vi "Write Subdiagram Labels.vi"(8 "Error In":errorcluster, 11 "DisableStructure In":refnum<vi>) -> (0 "Error Out":errorcluster, 3 "DisableStructure Out":refnum<vi>)   [LabVIEW 2017, in "Toolkit VIs.lvlib"]
uses:
  Toolkit VIs.lvlib
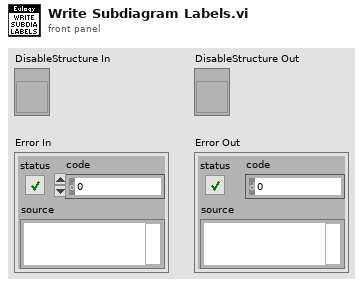
[diagram p1: front panel]
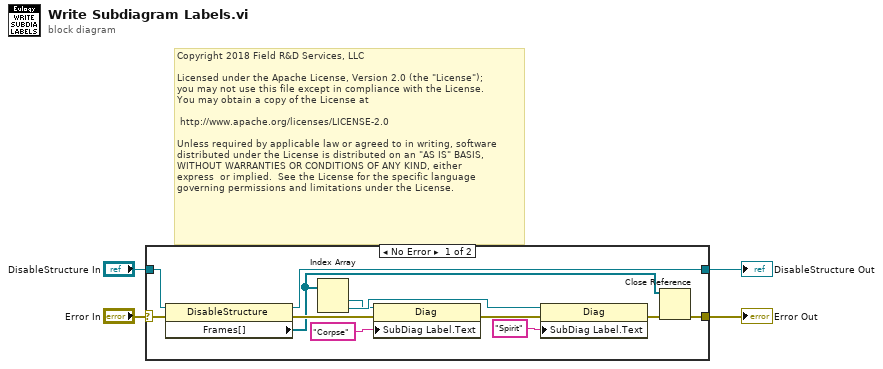
[diagram p0: block diagram]
diagram:
  # "Copyright 2018 Field R&D Services, LLC\n\nLicensed under the Apache License, Version 2.0 (the \"License\");\nyou may not use this file except in compliance with the License.\nYou may obtain a copy of the License at\n\n\thttp://www.apache.org/licenses/LICENSE-2.0\n\nUnless required by applicable law or agreed to in writing, software\ndistributed under the License is distributed on an \"AS IS\" BASIS,\nWITHOUT WARRANTIES OR CONDITIONS OF ANY KIND, either \nexpress  or implied.  See the License for the specific language \ngoverning permissions and limitations under the License."
  n1 = case shown="No Error" "Error In" {
    selector: "Error In" -> [w8 w17]
    tunnel: [w7 w17] -> w4
    tunnel: [w16 w18] -> w3
    tunnel: "DisableStructure In" -> [w10 w18]
    frame No Error {
      n2 = property class="DisableStructure"(reference=w10, error in=w8) -> (reference out=w16:refnum<vi>, error out=w9:errorcluster, "Frames[]"=w5:refnum<vi>[])
      n3 = Index Array(array=w5) -> (element #1=w12:refnum<vi>, element #2=w14:refnum<vi>)  [unwired: 2 in]
      n4 = property class="Diag"(reference=w12, error in=w9, "SubDiag Label.Text"="Corpse" ("Subdiagram Label.Text")) -> (error out=w11:errorcluster)  [unwired: 1 out]
      n5 = property class="Diag"(reference=w14, error in=w11, "SubDiag Label.Text"="Spirit" ("Subdiagram Label.Text")) -> (error out=w6:errorcluster)  [unwired: 1 out]
      n6 = Close Reference(reference=w5, error in (no error)=w6) -> (error out=w7:errorcluster)
    }
    frame Error {
    }
  }
  "Error Out" <- w4
  "DisableStructure Out" <- w3
